vi "niFpgaFFTStreamingProcessingControlUnit.vi"(0 "reset":bool, 2 "initial state":T1={"iteration count"=1024, "lty_count"=3099, "idxv"=FALSE, "os"=FALSE}, 12 "bitmask":u16=2047) -> (4 "stage switch":bool, 6 "twiddle address":u16, 8 "data index":u16, 10 "next state":enum8{"process", "idle"}(ring), 14 "state out":T2)   [LabVIEW 2017]
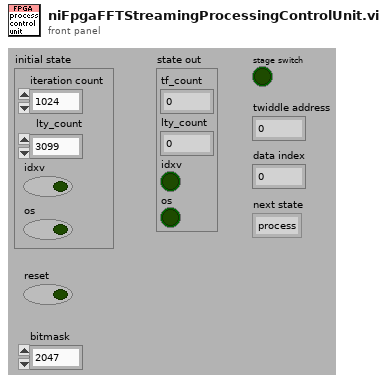
[diagram p1: front panel]
types:
  T1 = cluster{"iteration count":u16, "lty_count":u16, "idxv":bool, "os":bool}
  T2 = cluster{"tf_count":u16, "lty_count":u16, "idxv":bool, "os":bool}
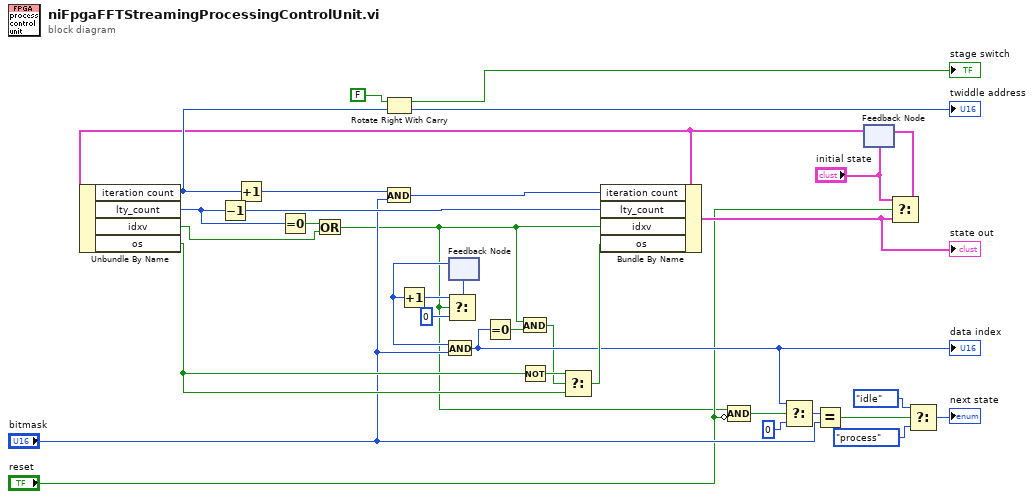
[diagram p0: block diagram]
diagram:
  n1 = feedback #1() -> (w10:u16)  [unwired: 1 out]
  n2 = Increment(x=w10) -> (x+1=w12:u16)
  n3 = And(x=w10, y="bitmask") -> (x .and. y?=w19:u16)
  "data index" <- w19
  n4 = Equal To 0?(x=w19) -> (x = 0?=w4:bool)
  n5 = feedback #2("initial state") -> (w15:T1)
  n6 = Unbundle By Name(w15) -> ("iteration count"=w30:u16, "lty_count"=w1:u16, "idxv"=w7:bool, "os"=w32:bool)
  n7 = Decrement(x=w1) -> (x-1=w13:u16)
  n8 = Increment(x=w30) -> (x+1=w27:u16)
  n9 = Equal To 0?(x=w1) -> (x = 0?=w8:bool)
  n10 = Or(x=w8, y=w7) -> (x .or. y?=w3:bool)
  n11 = Rotate Right With Carry(2:w30, 3:FALSE ("carry")) -> (0:→"twiddle address":u16, 1:→"stage switch":bool)
  n12 = And(x=w27, y="bitmask") -> (x .and. y?=w26:u16)
  n13 = Select(t=w12, s=w3, f=u16 0) -> (s? t:f=w11:u16)
  n14 = feedback-in #1(w11) -> ()
  n15 = And(x=w3, y=w4) -> (x .and. y?=w2:bool)
  n16 = Not(x=w32) -> (.not. x?=w33:bool)
  n17 = Select(t=w33, s=w2, f=w32) -> (s? t:f=w31:bool)
  n18 = Bundle By Name(cluster=w15, "iteration count"=w26, "lty_count"=w13, "idxv"=w3, "os"=w31) -> (w14:T1)
  "state out" <- w14
  n19 = Compound Arithmetic op=AND(w3, invert "reset") -> (w25:bool)
  n20 = Select(t=w19, s=w25, f=u16 0) -> (s? t:f=w23:u16)
  n21 = Equal?(x=w23, y="bitmask") -> (x = y?=w21:bool)
  n22 = Select(t="initial state", s="reset", f=w14) -> (s? t:f=w16:T1)
  n23 = feedback-in #2(w16) -> ()
  n24 = Select(t=enum8{"process", "idle"}."idle", s=w21, f=enum8{"process", "idle"}."process") -> (s? t:f=→"next state":enum8{"process", "idle"})
